vi "Init SPI.vi"(4 "CS Active Low (T)":bool=TRUE, 5 "CS GPIO (None)":i32=-1, 6 "SPI Config":T1={"Mode"=0, "Data Bits"=8, "MOSI Pin"=19, "MISO Pin"=16, "SCK Pin"=18}, 7 "Bus":u8, 8 "error in (no error)":errorcluster, 10 "Baud":u32=1000000 format="%.0p", 11 "VISA resource name in":refnum<visa-resource-name>) -> (0 "error out":errorcluster, 3 "VISA resource name":refnum<visa-resource-name>)   [LabVIEW 2024, in "CTIPicoVISA.lvlib"]
uses:
  SPI Config.ctl
  CTIPicoVISA.lvlib
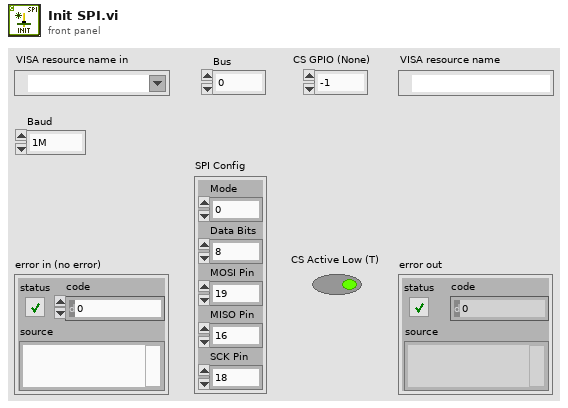
[diagram p1: front panel]
types:
  T1 = typedef "CTIPicoVISA.lvlib/SPI Config.ctl" = cluster{"Mode":u8, "Data Bits":u8, "MOSI Pin":u8, "MISO Pin":u8, "SCK Pin":u8}
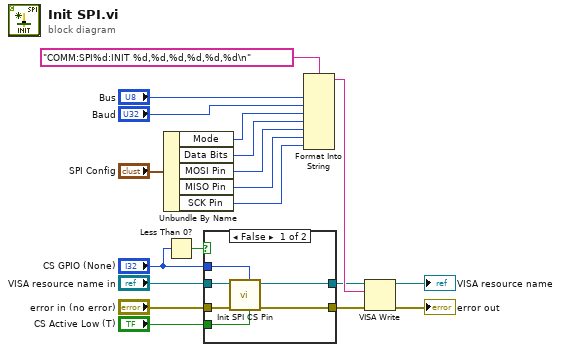
[diagram p0: block diagram]
diagram:
  n1 = Unbundle By Name("SPI Config") -> ("Mode"=w11:u8, "Data Bits"=w10:u8, "MOSI Pin"=w9:u8, "MISO Pin"=w8:u8, "SCK Pin"=w7:u8)
  n2 = Less Than 0?(x="CS GPIO (None)") -> (x < 0?=w1:bool)
  n3 = case shown="False" w1 {
    tunnel: "error in (no error)" -> [w25 w26]
    tunnel: [w24 w26] -> w6
    tunnel: "VISA resource name in" -> [w23 w27]
    tunnel: [w22 w27] -> w4
    tunnel: "CS GPIO (None)" -> [w21 _]
    tunnel: "CS Active Low (T)" -> [w20 _]
    frame False {
      n4 = call "Init SPI CS Pin.vi"("CS Active Low (T)"=w20, "CS GPIO"=w21, "error in (no error)"=w25, "VISA resource name in"=w23) -> ("error out"=w24:errorcluster, "VISA resource name"=w22:refnum<visa-resource-name>)  [unwired: 6 in]
    }
    frame True {
    }
  }
  n5 = Format Into String(format string="COMM:SPI%d:INIT %d,%d,%d,%d,%d,%d\n", "Bus", "Baud", w11, w10, w9, w8, w7) -> (resulting string=w14:string)  [unwired: 2 in, 1 out]
  n6 = VISA Write(VISA resource name=w4, write buffer=w14, error in (no error)=w6) -> (VISA resource name out=→"VISA resource name":refnum<visa-resource-name>, error out=→"error out":errorcluster)  [unwired: 1 out]
